vi "Signalverlaeufe mit Attributen erzeugen.vi"(8 "Log Sequence":i32[](array[numeric]), 9 "Messwerte":sgl[](array[numeric]), 10 "Namen":string[](array[string]), 11 "Zeitstempel":timestamp) -> (1 "Signalverläufe":waveform(dbl)[](array[waveform]))   [LabVIEW 2020, in "FT-IR.lvlib" / "TOOLweb Interface.lvlib" / "TOOLweb Interface Hilfs-VIs.lvlib"]
doc: "Setzt aus den Gas-Namen, dem Zeitstempel und den Messwerten für die einzelnen Gase NI-kompatible Signalverläufe zusammen, die als Attribut \"NI_ChannelName\" die Gasnamen automatisch als Plot-Namen an Diagramme übergeben können und eine korrekte Beschriftung der Zeitachse gewährleisten."
uses:
  TOOLweb Interface Hilfs-VIs.lvlib
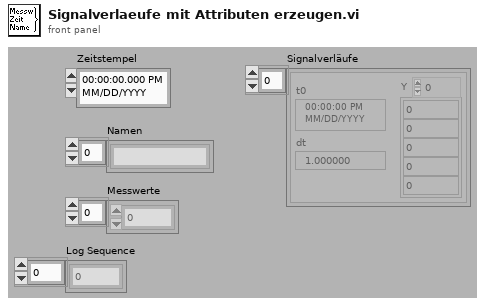
[diagram p1: front panel]
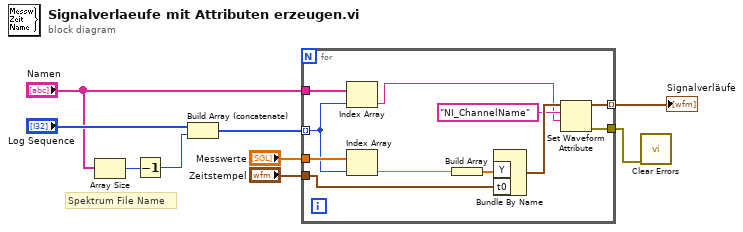
[diagram p0: block diagram]
diagram:
  # "Spektrum File Name"
  n1 = Array Size(array="Namen") -> (size(s)=w3:i32)
  n2 = Decrement(x=w3) -> (x-1=w2:i32)
  n3 = Build Array (concatenate)("Log Sequence", w2) -> (w1:i32[])
  n4 = for {
    tunnel: "Messwerte" -> [w12]
    tunnel: "Zeitstempel" -> [w19]
    tunnel: "Namen" -> [w14]
    tunnel: [w16] -> w9 mode=indexing
    tunnel: [w15] -> w6
    tunnel: w1 -> [w11] mode=indexing
    n5 = Index Array(array=w14, index=w11) -> (element=w13:string)
    n6 = Index Array(array=w12, index=w11) -> (element=w10:sgl)
    n7 = Build Array(w10) -> (w20:sgl[])
    n8 = Bundle By Name("Y"=w20, "t0"=w19) -> (w18:waveform(sgl))  [unwired: 1 out]
    n9 = Set Waveform Attribute(5:w13, 6:"NI_ChannelName" ("Name"), 7:w18) -> (0:w15:errorcluster, 3:w16:waveform(sgl))  [unwired: 1 in, 1 out]
  }
  "Signalverläufe" <- w9
  n10 = call <vilib>:"Clear Errors.vi"("error in (no error)"=w6) -> ()  [unwired: 5 in, 2 out]
